vi "Fire Quit Event.vi"(8 "error in (no error)":errorcluster, 10 "Force Quit?":bool, 11 "BaseSpecPage in":refnum<class "BaseSpecPage.lvclass">) -> (0 "error out":errorcluster, 2 "Quit OK?":bool, 3 "BaseSpecPage out":refnum<class "BaseSpecPage.lvclass">)   [LabVIEW 2016, in "BaseSpecPage.lvclass"]
uses:
  <resource>/dialog/NewProjectWizard/SpecPage/Base/BaseSpecPage.lvclass
  <resource>/dialog/NewProjectWizard/SpecPage/Base/BaseSpecPage.lvclass/BaseSpecPage.ctl
panel:
  # "For the base class, Force Quit? doesn't matter because the original Spec Pages always quit when it received a quit event."
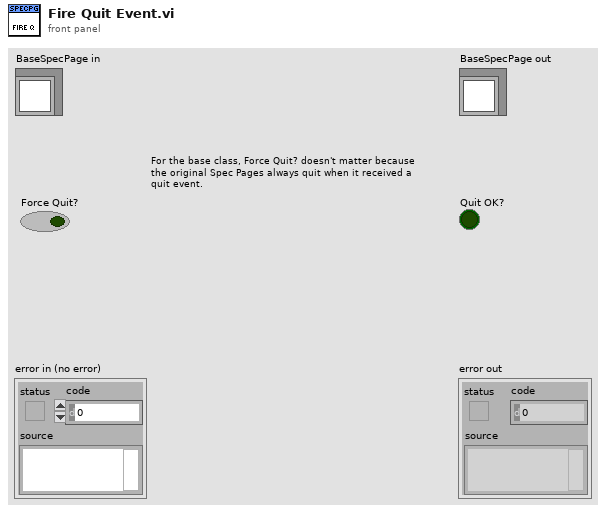
[diagram p1: front panel]
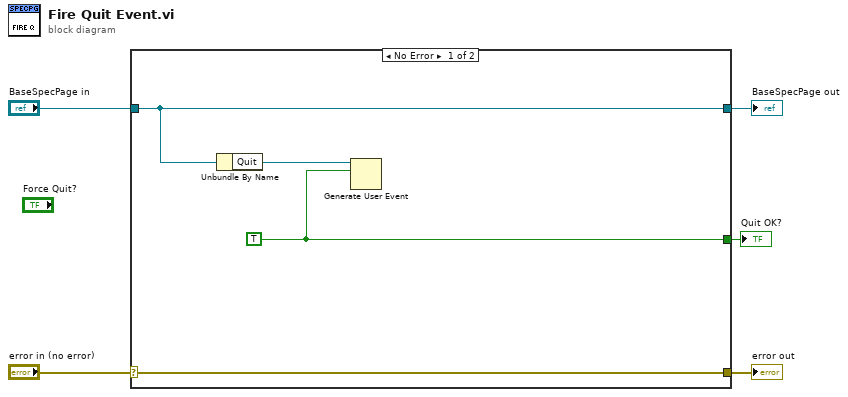
[diagram p0: block diagram]
diagram:
  n1 = case shown="No Error" "error in (no error)" {
    selector: "error in (no error)" -> [w6 w11]
    tunnel: [w6 w11] -> w4
    tunnel: [w9 w10] -> w2
    tunnel: "BaseSpecPage in" -> [w9 w10]
    tunnel: [w7 _] -> w1
    frame No Error {
      w7 = TRUE ("event data")
      n2 = Unbundle By Name(w9) -> ("Quit"=w8:refnum<user-event>)
      n3 = Generate User Event(user event=w8, event data cluster=w7) -> ()  [unwired: 2 in, 2 out]
    }
    frame Error {
    }
  }
  "error out" <- w4
  "BaseSpecPage out" <- w2
  "Quit OK?" <- w1
